vi "Write to log.vi"(8 "error in (no error)":errorcluster, 10 "Log":string, 11 "Logger in":refnum<class "Logger.lvclass">) -> (0 "error out":errorcluster, 3 "Logger out":refnum<class "Logger.lvclass">)   [LabVIEW 2017, in "Logger.lvclass"]
uses:
  Logger.lvclass
  Logger.lvclass/Logger.ctl
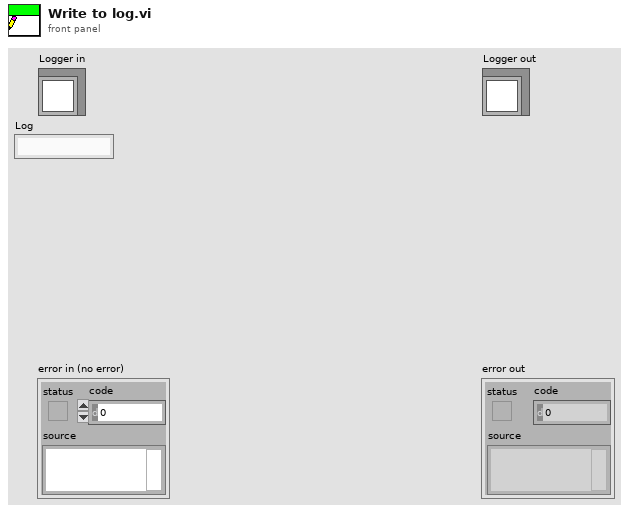
[diagram p1: front panel]
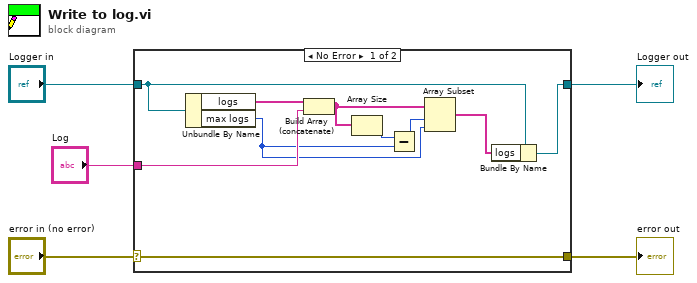
[diagram p0: block diagram]
diagram:
  n1 = case shown="No Error" "error in (no error)" {
    selector: "error in (no error)" -> [w15 w16]
    tunnel: [w15 w16] -> w4
    tunnel: [w14 w17] -> w2
    tunnel: "Logger in" -> [w13 w17]
    tunnel: "Log" -> [w11 _]
    frame No Error {
      n2 = Unbundle By Name(w13) -> ("logs"=w12:string[], "max logs"=w6:i64)
      n3 = Build Array (concatenate)(w12, w11) -> (w9:string[])
      n4 = Array Size(array=w9) -> (size(s)=w8:i32)
      n5 = Subtract(x=w8, y=w6) -> (x-y=w7:i64)
      n6 = Array Subset(array=w9, index=w7, length=w6) -> (w10:string[])
      n7 = Bundle By Name(cluster=w13, "logs"=w10) -> (w14:refnum<class "Logger.lvclass">)
    }
    frame Error {
    }
  }
  "error out" <- w4
  "Logger out" <- w2
